vi "LINX - Blink (Advanced).vi"() -> ()   [LabVIEW 2011, in "LVH-LINX.lvlib"]
doc: "Automatically blink and LED attached to a digital output channel of a LINX device."
uses:
  vi.lib/LabVIEW Hacker/LINX/LVH-LINX.lvlib
  vi.lib/LabVIEW Hacker/LINX/Public/Peripherals/Digital/Digital Write 1 Chan.vi
panel:
  out "LED Value":bool
  in  "Digital Output Channel":u8=13
  in  "Serial Port":refnum<visa-resource-name>
  out "Loop Rate (Hz)":u32
  in  "Stop Button":bool
  # "Circuit Schematic"
  # "LINX Device Settings"
  # "LED Value"
  # "Blink (Serial Interface)\n\nThis example demonstrates how to blink an LED on a LINX device connected to \nthe host computer using USB / Serial.\n\nInstructions\n1. Select the Serial Port associated with the LINX Device.\n2. Select the Digital Pin connected to the LED.\n3. Click the Run Arrow."
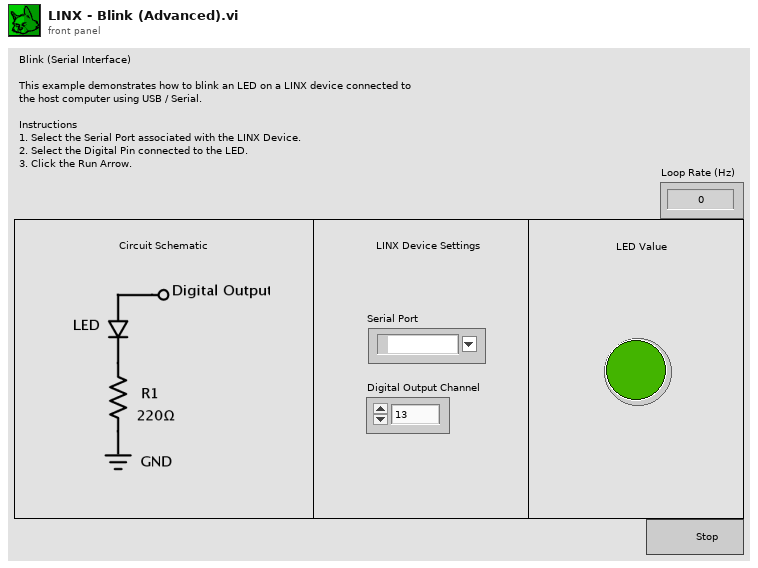
[diagram p1: front panel]
types:
  T1 = typedef "LVH-LINX.lvlib/LINX Ref.ctl" = cluster{"Platform":T2, "Interface":T3, "LINX Device Config":T4}
  T2 = typedef "LVH-LINX.lvlib/Platform.ctl" = enum16{"LINX", "myRIO"}
  T3 = typedef "LVH-LINX.lvlib/Interface.ctl" = enum16{"Serial", "TCP"}
  T4 = typedef "LVH-LINX.lvlib/Device.lvlib/LINX Device Config.ctl" = cluster{"Interface":T3, "COM Port":refnum<visa-resource-name>, "TCP Configuration":T5, "Device Family":u8, "Device ID":u8, "Device Name":string, "TCP Ref":refnum<k5>, "Channels":T6}
  T5 = typedef "LVH-LINX.lvlib/Device.lvlib/TCP Config.ctl" = cluster{"IP Address":string, "Port":u16}
  T6 = typedef "LVH-LINX.lvlib/Channels.ctl" = cluster{"DI":u8[], "DO":u8[], "AI":u8[], "AO":u8[], "PWM":u8[], "QE":u8[], "UART":u8[], "I2C 2":u8[], "SPI":u8[], "CAN":u8[], "Servo":u8[], "AI Ref (V)":dbl, "AO Ref (V)":dbl, "AO Resolution (Bits)":u8}
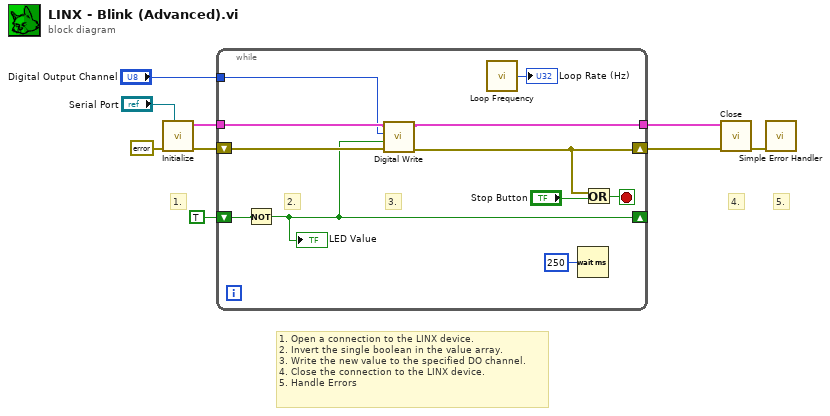
[diagram p0: block diagram]
diagram:
  # "1. Open a connection to the LINX device.\n2. Invert the single boolean in the value array.\n3. Write the new value to the specified DO channel.\n4. Close the connection to the LINX device.\n5. Handle Errors"
  # "5."
  # "4."
  # "1."
  n1 = call "Initialize.vi"("Serial Port"="Serial Port", "Error In"=errorcluster {"status"=FALSE, "code"=0, "source"=""}) -> ("Error Out"=w8:errorcluster, "LINX Ref"=w9:T1)  [unwired: 7 in, 1 out]
  n2 = while {
    tunnel: w9 -> [w17]
    tunnel: [w16] -> w7
    shift-right: [w14] -> w6
    shift-left: w8 -> [w15]
    shift-right: [w10] -> _
    shift-left: TRUE -> [w11]
    tunnel: "Digital Output Channel" -> [w12]
    stop <- w20 stop-if-true
    # "2."
    # "3."
    n3 = Not(x=w11) -> (.not. x?=w10:bool)
    "LED Value" <- w10
    n4 = call-poly "Digital Write.vi"("Error In"=w15, "Output Value"=w10, "DO Channel"=w12, "LINX Resource"=w17) -> ("Error Out"=w14:errorcluster, "LINX Resource"=w16:T1)  [unwired: 6 in]
    n5 = call "Loop Frequency.vi"() -> ("Loop Rate (Hz)"=→"Loop Rate (Hz)":u32)
    n6 = Wait (ms)(milliseconds to wait=u32 250) -> ()  [unwired: 1 out]
    n7 = Or(x=w14, y="Stop Button") -> (x .or. y?=w20:bool)
  }
  n8 = call "Close.vi"("Error In"=w6, "LINX Resource"=w7) -> ("Error Out"=w4:errorcluster)  [unwired: 8 in, 1 out]
  n9 = call <vilib>:"Simple Error Handler.vi"("error in (no error)"=w4) -> ()  [unwired: 4 in, 5 out]
